vi "data to file.vi"(8 "error in (no error)":errorcluster, 10 "Array":u64[](array[numeric]), 11 "Path":path) -> (0 "error out":errorcluster)   [LabVIEW 2021]
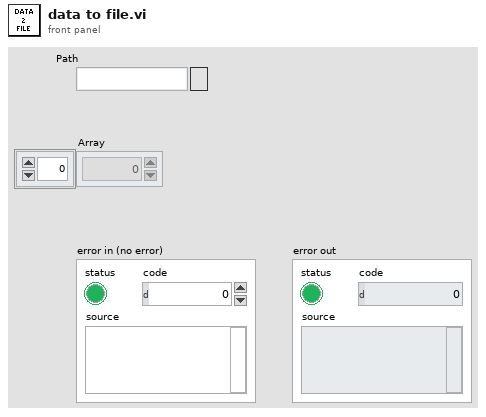
[diagram p1: front panel]
types:
  T1 = enum16{"open", "open or create", "create or replace", "create", "open (read-only)"}
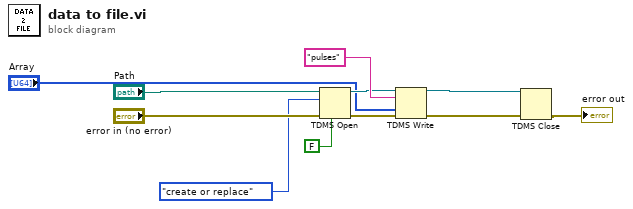
[diagram p0: block diagram]
diagram:
  n1 = TDMS Open(6:FALSE ("enable asynchronous? (T)"), 8:"error in (no error)", 10:T1."create or replace" ("operation (0:open)"), 11:"Path") -> (0:w3:errorcluster, 3:w5:refnum<k34>)  [unwired: 3 in]
  n2 = TDMS Write(0:w5, 5:"pulses" ("group name in (Untitled)"), 9:"Array", 11:w3) -> (4:w7:refnum<k34>, 15:w8:errorcluster)  [unwired: 2 in, 2 out]
  n3 = TDMS Close(8:w8, 11:w7) -> (0:→"error out":errorcluster)  [unwired: 1 out]
